vi "HackRF_SetFreq_Sample.vi"(8 "error in (no error)":errorcluster, 9 "FilterBandwidthHz":dbl=-1.0 format="%#_6p", 10 "SampleFreqHz":dbl format="%#_6p", 11 "HackRF in":T1) -> (0 "error out":errorcluster, 3 "HackRF out":T1)   [LabVIEW 2020]
doc: "Set sample frequency in MHz"
uses:
  HackRF_Ref.ctl
  D:/Programming/Labview/HackRF/HackRF_Lib/NetHackrf.dll
  NetHackrf.dll
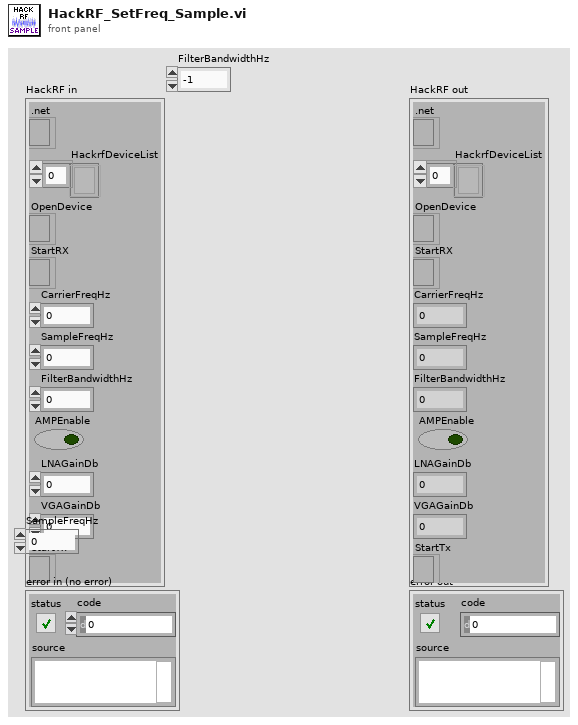
[diagram p1: front panel]
types:
  T1 = typedef "HackRF_Ref.ctl" = cluster{".net":refnum<k24>, "HackrfDeviceList":refnum<k24>[], "OpenDevice":refnum<k24>, "StartRX":refnum<k24>, "CarrierFreqHz":dbl, "SampleFreqHz":dbl, "FilterBandwidthHz":dbl, "AMPEnable":bool, "LNAGainDb":dbl, "VGAGainDb":dbl, "StartTx":refnum<k24>}
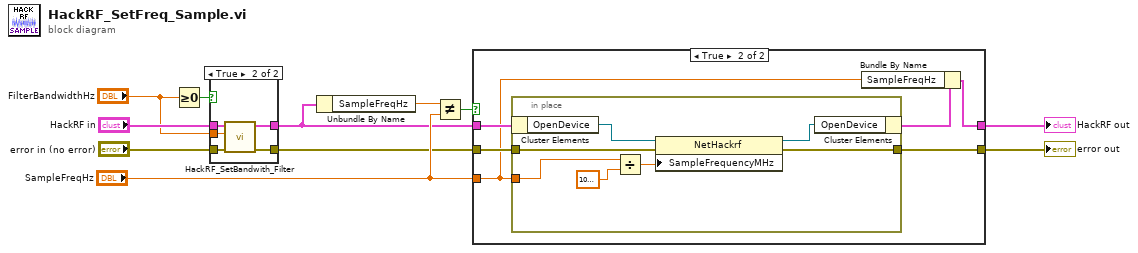
[diagram p0: block diagram]
diagram:
  n1 = Greater Or Equal To 0?(x="FilterBandwidthHz") -> (x >= 0?=w1:bool)
  n2 = case shown="True" w1 {
    tunnel: "error in (no error)" -> [w13 w18]
    tunnel: "HackRF in" -> [w12 w17]
    tunnel: [w13 w16] -> w4
    tunnel: [w12 w15] -> w3
    tunnel: "FilterBandwidthHz" -> [_ w14]
    frame False {
    }
    frame True {
      n3 = call "HackRF_SetBandwith_Filter.vi"("error in (no error)"=w18, "FilterBandwidth"=w14, "HackRF in"=w17) -> ("error out"=w16:errorcluster, "HackRF out"=w15:T1)  [unwired: 7 in]
    }
  }
  n4 = Unbundle By Name(w3) -> ("SampleFreqHz"=w9:dbl)
  n5 = Not Equal?(x=w9, y="SampleFreqHz") -> (x != y?=w7:bool)
  n6 = case shown="True" w7 {
    tunnel: w4 -> [w20 w26]
    tunnel: [w20 w25] -> w11
    tunnel: [w19 w22] -> w10
    tunnel: w3 -> [w19 w24]
    tunnel: "SampleFreqHz" -> [_ w21]
    frame False {
    }
    frame True {
      n7 = in-place {
        in-place-border: w26 -> [w31]
        in-place-border: [w30] -> w25
        in-place-border: w21 -> [w28]
        n8 = in-place-cluster #1(w24) -> ("OpenDevice"=w33:refnum<k24>)
        n9 = Divide(x=w28, y=1000000.0) -> (x/y=w29:dbl)
        n10 = property class="NetHackrf"(reference=w33, error in=w31, "SampleFrequencyMHz"=w29) -> (reference out=w32:refnum<k24>, error out=w30:errorcluster)
        n11 = in-place-cluster #1("OpenDevice"=w32) -> (w23:T1)
      }
      n12 = Bundle By Name(cluster=w23, "SampleFreqHz"=w21) -> (w22:T1)
    }
  }
  "error out" <- w11
  "HackRF out" <- w10
